vi "check_win.vi"(8 "check against":string, 11 "Array":string[](array[string])) -> (2 "result":bool)   [LabVIEW 2026]
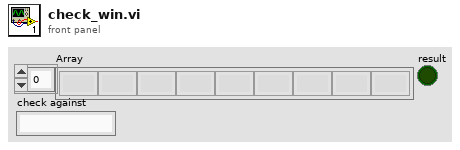
[diagram p1: front panel]
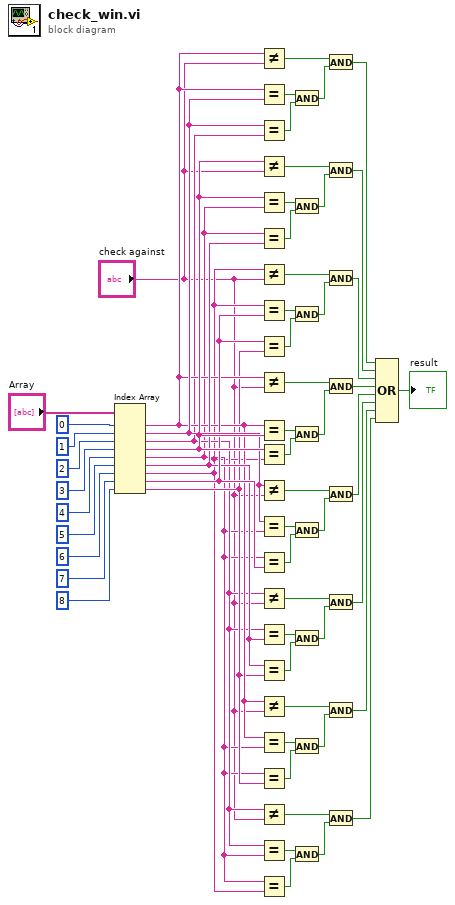
[diagram p0: block diagram]
diagram:
  n1 = Index Array(array="Array", index #1=0 ("index"), index #2=1 ("index"), index #3=2 ("index"), index #4=3 ("index"), index #5=4 ("index"), index #6=5 ("index"), index #7=6 ("index"), index #8=7 ("index"), index #9=8 ("index")) -> (element #1=w13:string, element #2=w26:string, element #3=w6:string, element #4=w32:string, element #5=w5:string, element #6=w19:string, element #7=w4:string, element #8=w25:string, element #9=w12:string)
  n2 = Not Equal?(x=w13, y="check against") -> (x != y?=w47:bool)
  n3 = Equal?(x=w13, y=w26) -> (x = y?=w50:bool)
  n4 = Equal?(x=w26, y=w6) -> (x = y?=w51:bool)
  n5 = Not Equal?(x=w32, y="check against") -> (x != y?=w43:bool)
  n6 = Equal?(x=w32, y=w5) -> (x = y?=w49:bool)
  n7 = Equal?(x=w5, y=w19) -> (x = y?=w48:bool)
  n8 = Not Equal?(x=w4, y="check against") -> (x != y?=w42:bool)
  n9 = Equal?(x=w4, y=w25) -> (x = y?=w41:bool)
  n10 = Equal?(x=w25, y=w12) -> (x = y?=w40:bool)
  n11 = Not Equal?(x=w13, y="check against") -> (x != y?=w34:bool)
  n12 = Equal?(x=w13, y=w32) -> (x = y?=w35:bool)
  n13 = Equal?(x=w32, y=w4) -> (x = y?=w36:bool)
  n14 = Not Equal?(x=w26, y="check against") -> (x != y?=w28:bool)
  n15 = Equal?(x=w26, y=w5) -> (x = y?=w29:bool)
  n16 = Equal?(x=w5, y=w25) -> (x = y?=w30:bool)
  n17 = Not Equal?(x=w6, y="check against") -> (x != y?=w21:bool)
  n18 = Equal?(x=w6, y=w19) -> (x = y?=w22:bool)
  n19 = Equal?(x=w19, y=w12) -> (x = y?=w23:bool)
  n20 = Not Equal?(x=w13, y="check against") -> (x != y?=w15:bool)
  n21 = Equal?(x=w13, y=w5) -> (x = y?=w16:bool)
  n22 = Equal?(x=w5, y=w12) -> (x = y?=w17:bool)
  n23 = Not Equal?(x=w6, y="check against") -> (x != y?=w8:bool)
  n24 = Equal?(x=w6, y=w5) -> (x = y?=w9:bool)
  n25 = Equal?(x=w5, y=w4) -> (x = y?=w10:bool)
  n26 = And(x=w50, y=w51) -> (x .and. y?=w46:bool)
  n27 = And(x=w49, y=w48) -> (x .and. y?=w45:bool)
  n28 = And(x=w41, y=w40) -> (x .and. y?=w44:bool)
  n29 = And(x=w35, y=w36) -> (x .and. y?=w33:bool)
  n30 = And(x=w29, y=w30) -> (x .and. y?=w27:bool)
  n31 = And(x=w22, y=w23) -> (x .and. y?=w20:bool)
  n32 = And(x=w16, y=w17) -> (x .and. y?=w14:bool)
  n33 = And(x=w9, y=w10) -> (x .and. y?=w7:bool)
  n34 = And(x=w47, y=w46) -> (x .and. y?=w39:bool)
  n35 = And(x=w43, y=w45) -> (x .and. y?=w38:bool)
  n36 = And(x=w42, y=w44) -> (x .and. y?=w37:bool)
  n37 = And(x=w34, y=w33) -> (x .and. y?=w31:bool)
  n38 = And(x=w28, y=w27) -> (x .and. y?=w24:bool)
  n39 = And(x=w21, y=w20) -> (x .and. y?=w18:bool)
  n40 = And(x=w15, y=w14) -> (x .and. y?=w11:bool)
  n41 = And(x=w8, y=w7) -> (x .and. y?=w3:bool)
  n42 = Compound Arithmetic op=OR(w39, w38, w37, w31, w24, w18, w11, w3) -> (→"result":bool)
